vi "Update DUT Status.vi"(8 "error in (no error)":errorcluster, 10 "String":string, 11 "Device Under Test In":refnum<class "Device Under Test.lvclass">) -> (0 "error out":errorcluster, 3 "Device Under Test Out":refnum<class "Device Under Test.lvclass">)   [LabVIEW 2020, in "Device Under Test.lvclass"]
uses:
  Device Under Test.lvclass
  C:/Program Files (x86)/National Instruments/LabVIEW 2020/vi.lib/Asteme/Triarc Framework/Process/Process.lvclass
  <vilib>/Asteme/Triarc Framework/Process/Process.lvclass/Process.ctl
  <vilib>/Utility/error.llb/Clear Errors.vi
  <vilib>/Asteme/Triarc Framework/Process/Process.lvclass
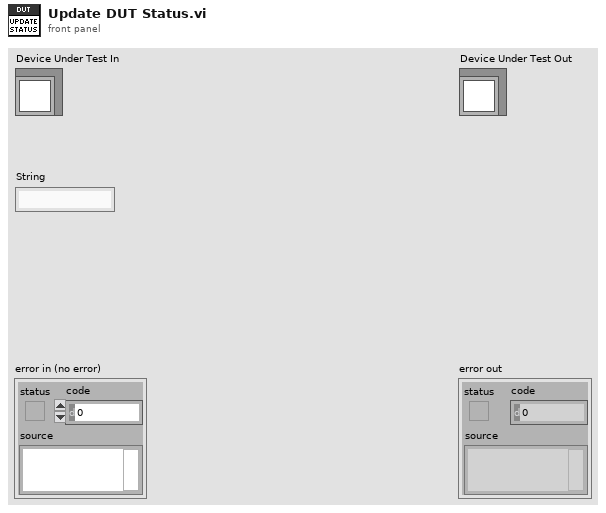
[diagram p1: front panel]
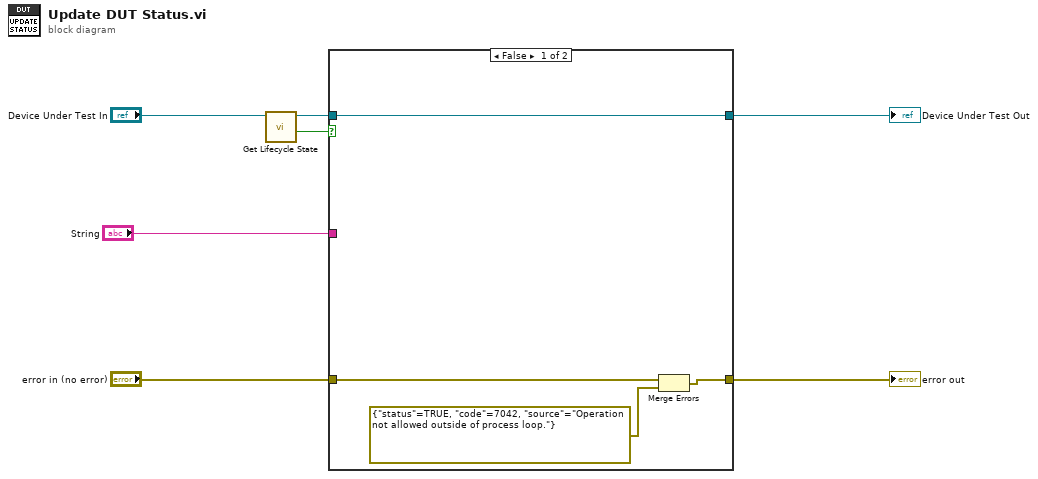
[diagram p0: block diagram]
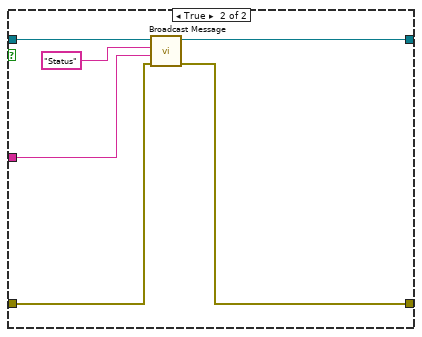
[diagram p2: hidden frame]
diagram:
  n1 = call <vilib>:"Get Lifecycle State.vi"("Process In"="Device Under Test In") -> ("In Process Loop?"=w1:bool, "Process Out"=w4:refnum<class "Device Under Test.lvclass">)  [unwired: 7 in, 2 out]
  n2 = case shown="False" w1 {
    tunnel: "error in (no error)" -> [w10 w17]
    tunnel: [w9 w16] -> w5
    tunnel: w4 -> [w11 w15]
    tunnel: [w11 w14] -> w3
    tunnel: "String" -> [_ w12]
    frame False {
      n3 = Merge Errors(w10, errorcluster {"status"=TRUE, "code"=7042, "source"="Operation not allowed outside of process loop."} ("error in")) -> (w9:errorcluster)
    }
    frame True {
      n4 = call-dynamic "Broadcast Message.vi"("error in (no error)"=w17, "Message Data"=w12, "Message"="Status", "Rig Process In"=w15) -> ("error out"=w16:errorcluster, "Rig Process Out"=w14:refnum<class "Device Under Test.lvclass">)  [unwired: 6 in]
    }
  }
  "error out" <- w5
  "Device Under Test Out" <- w3
